vi "XML Main.vi"(8 "Error In":errorcluster, 11 "path to XML document 2":path caption="path to XML document") -> (0 "Error Out":errorcluster, 3 "Expressions":string[][](array[string]))   [LabVIEW 2014]
uses:
  Type Definitions/XML Data Type.ctl
  <vilib>/xml/Close Reference(Node).vi
  <vilib>/xml/NI_XML.lvlib
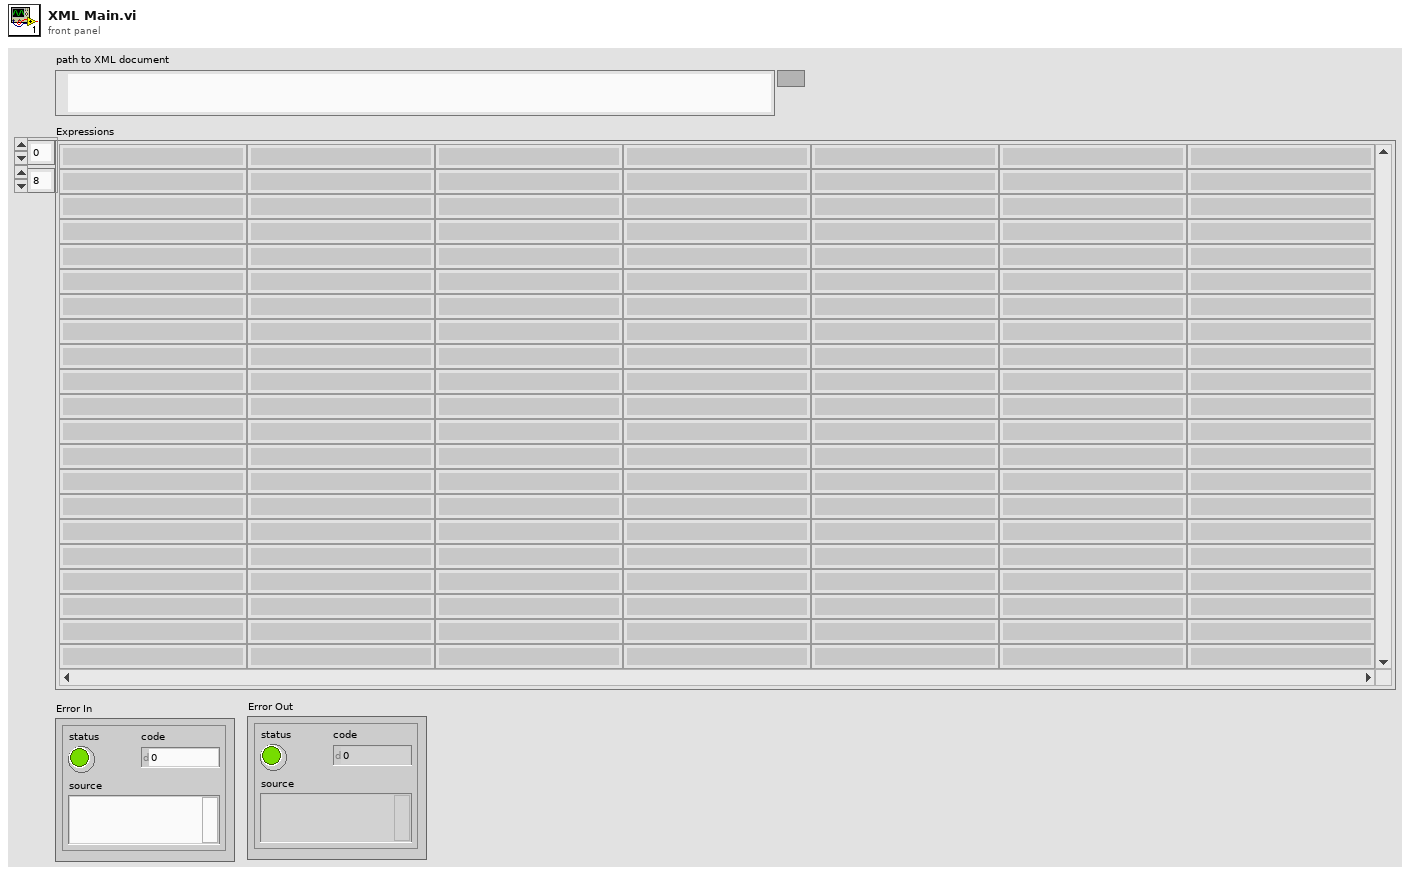
[diagram p1: front panel]
types:
  T1 = typedef "XML Data Type.ctl" = enum16{"Name", "Value"}
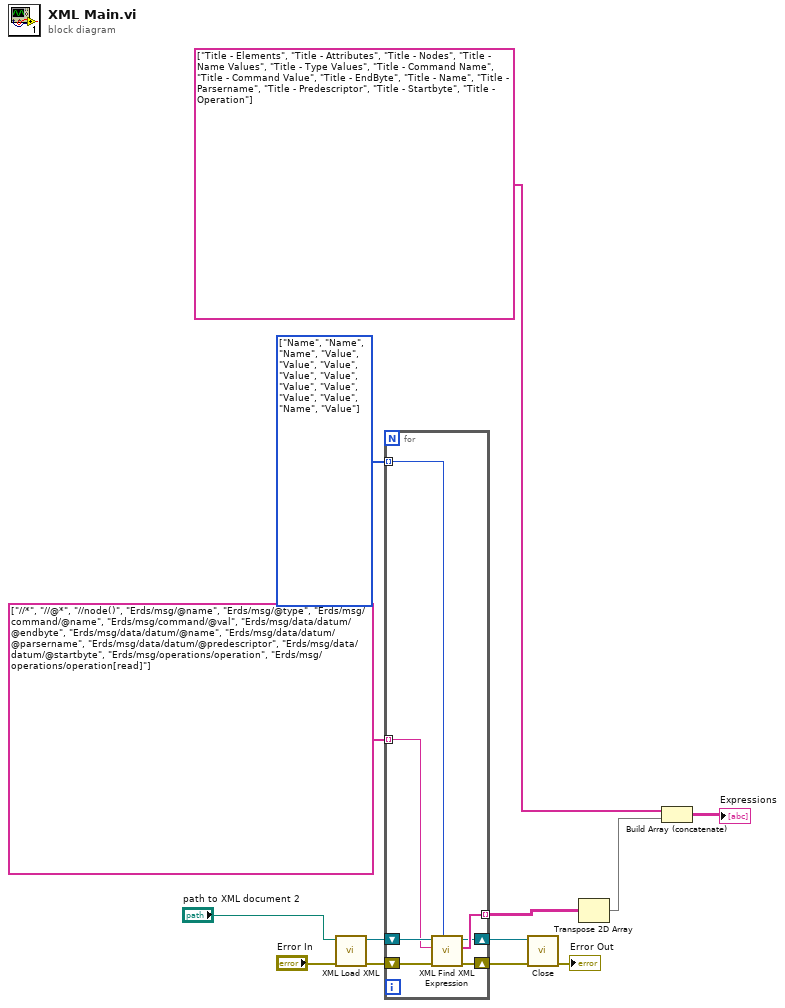
[diagram p0: block diagram]
diagram:
  w10 = T1[] [enum."Name", enum."Name", enum."Name", enum."Value", enum."Value", enum."Value", enum."Value", enum."Value", enum."Value", enum."Value", enum."Value", enum."Value", enum."Name", enum."Value"] items=["Name", "Value"]
  n1 = call "XML Load XML.vi"("Error In"="Error In", "path to XML document in"="path to XML document 2") -> ("Error Out"=w5:errorcluster, "Refnum out"=w12:refnum<k20>)  [unwired: 8 in]
  n2 = for {
    tunnel: string[] ["//*", "//@*", "//node()", "Erds/msg/@name", "Erds/msg/@type", "Erds/msg/command/@name", "Erds/msg/command/@val", "Erds/msg/data/datum/@endbyte", "Erds/msg/data/datum/@name", "Erds/msg/data/datum/@parsername", "Erds/msg/data/datum/@predescriptor", "Erds/msg/data/datum/@startbyte", "Erds/msg/operations/operation", "Erds/msg/operations/operation[read]"] -> [w19] mode=indexing
    tunnel: [w18] -> w4 mode=indexing
    tunnel: w10 -> [w17] mode=indexing
    shift-right: [w16] -> w8
    shift-left: w12 -> [w20]
    shift-right: [w15] -> w9
    shift-left: w5 -> [w14]
    n3 = call "XML Find XML Expression.vi"("Data Type"=w17, "error in (no error)"=w14, "XPath expression"=w19, "Refnum in"=w20) -> ("error out"=w15:errorcluster, "Expressions"=w18:string[], "Refnum out"=w16:refnum<k20>)  [unwired: 5 in]
  }
  n4 = call-poly <vilib>:"Close.vi"("error in (no error)"=w9, "node"=w8) -> ("error out"=→"Error Out":errorcluster)  [unwired: 7 in]
  n5 = Transpose 2D Array(2D array=w4) -> (transposed array=w2:string[][])
  n6 = Build Array (concatenate)(string[] ["Title - Elements", "Title - Attributes", "Title - Nodes", "Title - Name Values", "Title - Type Values", "Title - Command Name", "Title - Command Value", "Title - EndByte", "Title - Name", "Title - Parsername", "Title - Predescriptor", "Title - Startbyte", "Title - Operation"], w2) -> (→"Expressions":string[][])
